vi "CutZeroRows2.vi"(1 "# Cols":i32, 2 "# Rows":i32, 3 "Array IN":dbl[][](array[numeric])) -> (0 "Array OUT":dbl[][](array[numeric]))   [LabVIEW 2017]
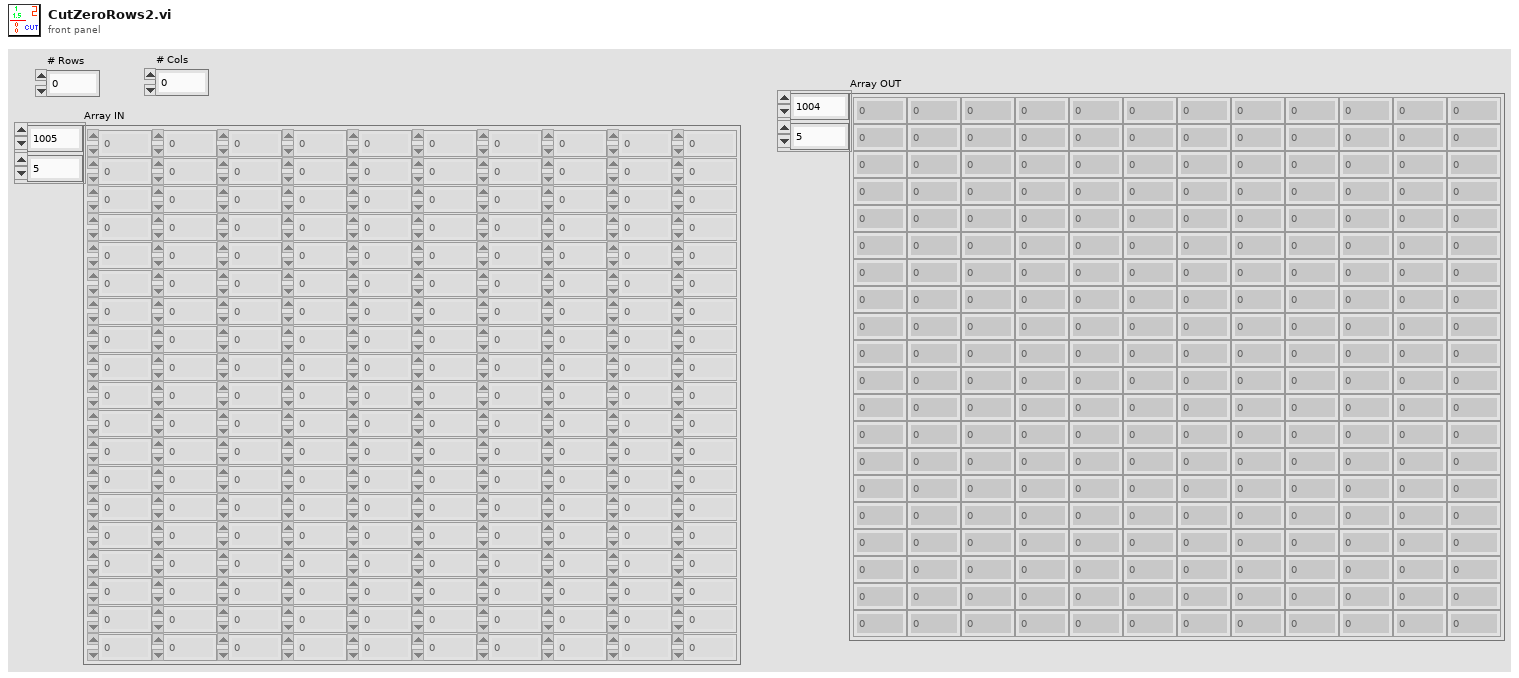
[diagram p1: front panel]
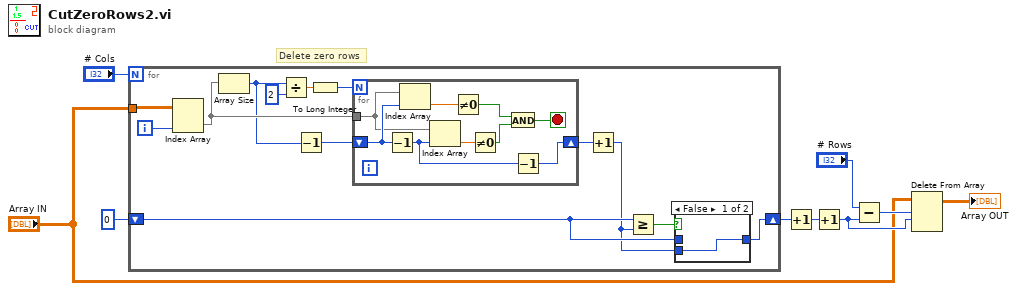
[diagram p0: block diagram]
diagram:
  # "Delete zero rows"
  n1 = for {
    N: "# Cols" -> [_]
    tunnel: "Array IN" -> [w22]
    shift-right: [w17] -> w5
    shift-left: 0 -> [w18]
    i -> [w21]
    n2 = Index Array(array=w22, index (col)=w21) -> (element=w20:dbl[])  [unwired: 1 in]
    n3 = Array Size(array=w20) -> (size(s)=w13:i32)
    n4 = Divide(x=w13, y=2) -> (x/y=w15:dbl)
    n5 = Decrement(x=w13) -> (x-1=w12:i32)
    n6 = To Long Integer(number=w15) -> (32bit integer=w14:i32)
    n7 = for {
      N: w14 -> [_]
      tunnel: w20 -> [w32]
      shift-right: [w25] -> w11
      shift-left: w12 -> [w33]
      stop <- w27 stop-if-true
      n8 = Decrement(x=w33) -> (x-1=w26:i32)
      n9 = Index Array(array=w32, index=w33) -> (element=w31:dbl)
      n10 = Index Array(array=w32, index=w26) -> (element=w30:dbl)
      n11 = Not Equal To 0?(x=w31) -> (x != 0?=w29:bool)
      n12 = Not Equal To 0?(x=w30) -> (x != 0?=w28:bool)
      n13 = And(x=w29, y=w28) -> (x .and. y?=w27:bool)
      n14 = Decrement(x=w26) -> (x-1=w25:i32)
    }
    n15 = Increment(x=w11) -> (x+1=w10:i32)
    n16 = Greater Or Equal?(x=w18, y=w10) -> (x >= y?=w19:bool)
    n17 = case shown="False" w19 {
      tunnel: w18 -> [_ w24]
      tunnel: [w23 w24] -> w17
      tunnel: w10 -> [w23 _]
      frame False {
      }
      frame True {
      }
    }
  }
  n18 = Increment(x=w5) -> (x+1=w4:i32)
  n19 = Increment(x=w4) -> (x+1=w3:i32)
  n20 = Subtract(x="# Rows", y=w3) -> (x-y=w8:i32)
  n21 = Delete From Array(array="Array IN", length=w8, index (row)=w3) -> (array with subset deleted=→"Array OUT":dbl[][])  [unwired: 1 in, 1 out]
